vi "isQueueTcpClientFull.vi"(8 "error in (no error)":errorcluster, 10 "queueName":T1(ring), 11 "tcpServer in":refnum<class "TcpServer.lvclass">) -> (0 "error out":errorcluster, 2 "queueFull":bool, 3 "tcpServer out":refnum<class "TcpServer.lvclass">)   [LabVIEW 2018, in "TcpServer.lvclass"]
doc: "Check if queue is full to send or receive telemetry. This returns TRUE if queue is full and FALSE if not. Use the queueName enum control to select queueTcpClientFromDds or queueTcpClient options.\n\nNote: this function will not handle any error internally, so the user must handle the errors when call it."
uses:
  TcpServer.lvclass
  TcpServer.lvclass/TcpServer.ctl
  TcpServerTel/TcpServerTel.lvclass
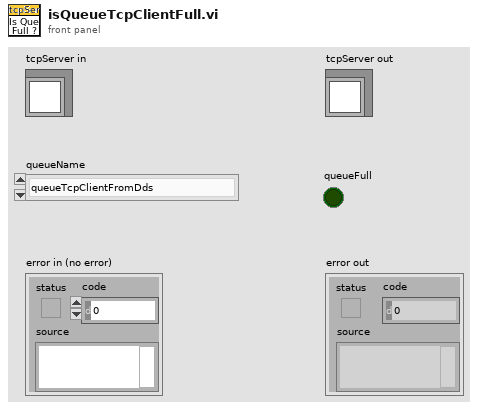
[diagram p1: front panel]
types:
  T1 = enum16{"queueTcpClientFromDds", "queueTcpClient"}
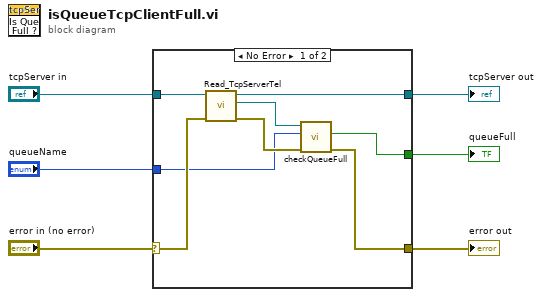
[diagram p0: block diagram]
diagram:
  n1 = case shown="No Error" "error in (no error)" {
    selector: "error in (no error)" -> [w13 w16]
    tunnel: [w10 w16] -> w5
    tunnel: "tcpServer in" -> [w14 w15]
    tunnel: [w9 w15] -> w3
    tunnel: [w8 _] -> w2
    tunnel: "queueName" -> [w7 _]
    frame No Error {
      n2 = call "Read_TcpServerTel.vi"("error in (no error)"=w13, "TcpServer in"=w14) -> ("error out"=w11:errorcluster, "TcpServerTel.lvclass"=w12:refnum<class "TcpServerTel.lvclass">, "TcpServer out"=w9:refnum<class "TcpServer.lvclass">)  [unwired: 7 in]
      n3 = call "checkQueueFull.vi"("error in (no error)"=w11, "queueName"=w7, "tcpServerTel in"=w12) -> ("error out"=w10:errorcluster, "queueFull"=w8:bool)  [unwired: 6 in, 1 out]
    }
    frame Error {
    }
  }
  "error out" <- w5
  "tcpServer out" <- w3
  "queueFull" <- w2
